vi "To AUT Error.vi"(7 "Enqueuer ID":string, 8 "error in (no error)":errorcluster, 9 "Error to Send":errorcluster, 11 "Test Harness in":refnum<class "User Interface Tester.lvclass">) -> (0 "error out":errorcluster, 3 "Test Harness out":refnum<class "User Interface Tester.lvclass">)   [LabVIEW 2020, in "User Interface Tester.lvlib" / "User Interface Tester.lvclass"]
uses:
  User Interface Tester.lvclass
  User Interface Tester.lvclass/User Interface Tester.ctl
  <vilib>/ActorFramework/Report Error Msg/Report Error Msg.lvclass/Report Error Msg.ctl
  <vilib>/ActorFramework/Message Enqueuer/Message Enqueuer.lvclass/Message Enqueuer.ctl
  <vilib>/ActorFramework/Message Enqueuer/Enqueue.vi
  <vilib>/ActorFramework/Report Error Msg/Report Error Msg.lvclass
  C:/Program Files (x86)/National Instruments/LabVIEW 2020/vi.lib/ActorFramework/Message/Message.lvclass
  <vilib>/ActorFramework/Message Priority Queue/Priority Enqueue.vi
  <vilib>/SAS/Actor Tester/Enqueuer Manager/SAS_AFTester_Enqueuer Manager.lvclass
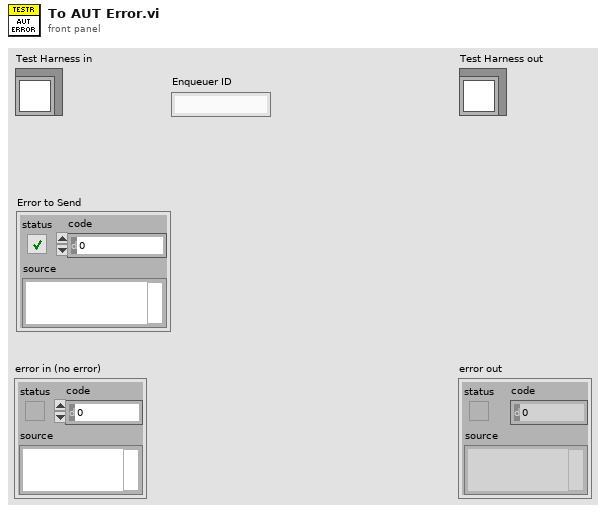
[diagram p1: front panel]
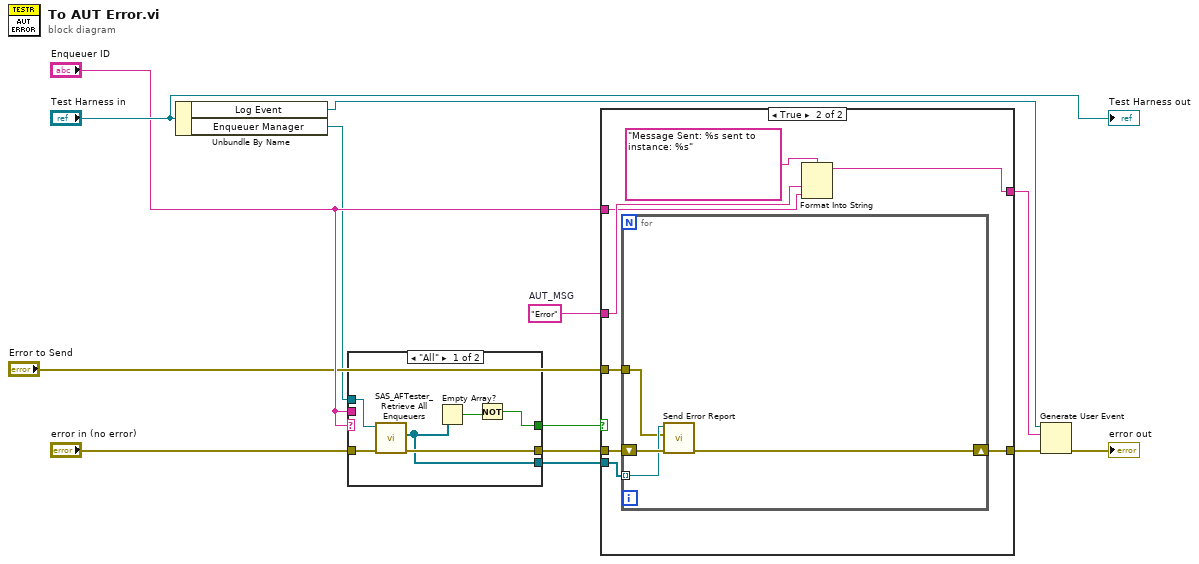
[diagram p0: block diagram]
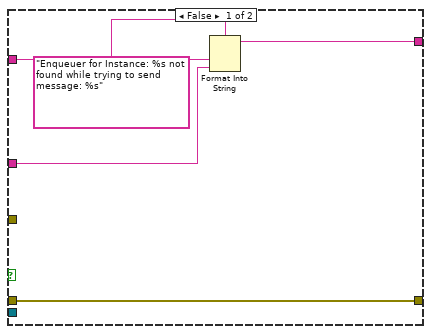
[diagram p2: hidden frame]
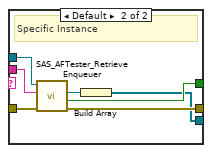
[diagram p3: hidden frame]
diagram:
  w2 = "Error"  # AUT_MSG
  n1 = Unbundle By Name("Test Harness in") -> ("Log Event"=w4:refnum<user-event>, "Enqueuer Manager"=w8:refnum<class "SAS_AFTester_Enqueuer Manager.lvclass">)
  n2 = case shown="\"All\"" "Enqueuer ID" {
    tunnel: w8 -> [w19 w26]
    tunnel: "error in (no error)" -> [w18 w25]
    tunnel: [w17 w24] -> w7
    tunnel: "Enqueuer ID" -> [_ w23]
    tunnel: [w16 w20] -> w5
    tunnel: [w14 w21] -> w6
    frame "All" {
      n3 = call <vilib>:"SAS_AFTester_Retrieve All Enqueuers.vi"("error in (no error)"=w18, "Enqueuer Manager in"=w19) -> ("error out"=w17:errorcluster, "Enqueuers"=w16:refnum<class "Message Enqueuer.lvclass">[])  [unwired: 7 in, 1 out]
      n4 = Empty Array?(array=w16) -> (empty?=w15:bool)
      n5 = Not(x=w15) -> (.not. x?=w14:bool)
    }
    frame Default {
      # "Specific Instance"
      n6 = call <vilib>:"SAS_AFTester_Retrieve Enqueuer.vi"("error in (no error)"=w25, "Enqueuer ID"=w23, "Enqueuer Manager in"=w26) -> ("error out"=w24:errorcluster, "Found?"=w21:bool, "Message Enqueuer"=w22:refnum<class "Message Enqueuer.lvclass">)  [unwired: 5 in, 1 out]
      n7 = Build Array(w22) -> (w20:refnum<class "Message Enqueuer.lvclass">[])
    }
  }
  n8 = case shown="True" w6 {
    tunnel: w7 -> [w31 w39]
    tunnel: w5 -> [_ w38]
    tunnel: [w31 w37] -> w3
    tunnel: w2 -> [w29 w34]
    tunnel: "Enqueuer ID" -> [w28 w33]
    tunnel: [w27 w35] -> w1
    tunnel: "Error to Send" -> [_ w32]
    frame False {
      n9 = Format Into String(format string="Enqueuer for Instance: %s not found while trying to send message: %s", w28, w29) -> (resulting string=w27:string)  [unwired: 2 in, 1 out]
    }
    frame True {
      n10 = for {
        tunnel: w38 -> [w42] mode=indexing
        shift-right: [w41] -> w37
        shift-left: w39 -> [w43]
        tunnel: w32 -> [w40]
        n11 = call <vilib>:"Send Error Report.vi"("error in (no error)"=w43, "Error From Sender"=w40, "Message Enqueuer"=w42) -> ("error out"=w41:errorcluster)  [unwired: 8 in]
      }
      n12 = Format Into String(format string="Message Sent: %s sent to instance: %s", w34, w33) -> (resulting string=w35:string)  [unwired: 2 in, 1 out]
    }
  }
  n13 = Generate User Event(user event=w4, event data cluster=w1, error in=w3) -> (error out=→"error out":errorcluster)  [unwired: 1 in, 1 out]
  "Test Harness out" <- "Test Harness in"
